vi "4145 Send Message.vi"(4 "source IN":string, 5 "status IN":bool[](array[boolean]), 7 "timeout ms":u32=25000, 8 "error in":T2, 9 "write mode (set END:0)":i32(ring) items=["send EOI with last character of string", "append CR to string and send EOI with CR", "append LF to string and send EOI with LF", "append CR LF to string and send EOI with LF", "append CR to string but do not send EOI", "append LF to string but do not send EOI", "append CR LF to string but do not send EOI", "do not send EOI"], 10 "write buffer IN":string, 11 "4145_GPIB_COM_IN":T1={"Address_string"="17", "timeout ms"=25000, "Terminator"=",", "LoggerQueue"=refnum}) -> (0 "error out":T2, 1 "status OUT":bool[](array[boolean]), 2 "byte count OUT":i32, 3 "4145_GPIB_COM_OUT":T1={"Address_string"="17", "timeout ms"=25000, "Terminator"=",", "LoggerQueue"=refnum})   [LabVIEW 2014]
doc: "Sends a string to a message based VXI instrument. In order to communicate with an instrument, you must first open the instrument by running the Open VXI Instrument or running the initialize VI (initialize VIs call the Open VXI Instrument in their block diagram). Use the instrument ID generated by the Open VXI Instrument to address the specific instrument, then set the write mode and enter the string to send. If a write error occurs, error code 1230 is returned. If you fail to open the instrument, error code 1232 is returned."
uses:
  typedef/4145_GPIB_Com.ctl
  typedef/4145_que_msg.ctl
  typedef/4145 command enum.ctl
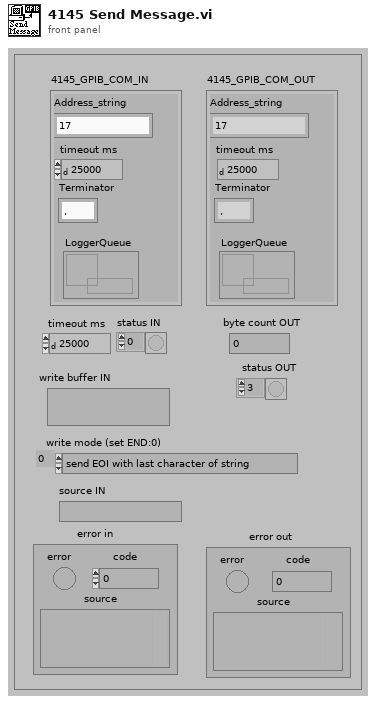
[diagram p1: front panel]
types:
  T1 = typedef "4145_GPIB_Com.ctl" = cluster{"Address_string":string, "timeout ms":u32, "Terminator":string, "LoggerQueue":refnum<queue>}
  T2 = cluster{"error":bool, "code":i32, "source":string}
  T3 = typedef "4145 command enum.ctl" = enum16{"DEFAULT", "INFORMATION", "ERROR", "STATUS", "CAUTION", "WARNING", "OFFLINE", "STOP"}
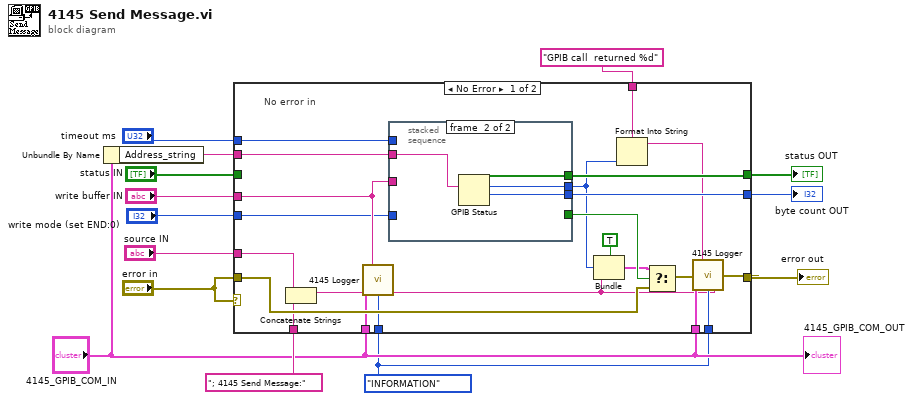
[diagram p0: block diagram]
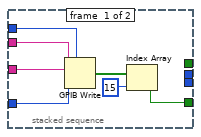
[diagram p2: hidden frame]
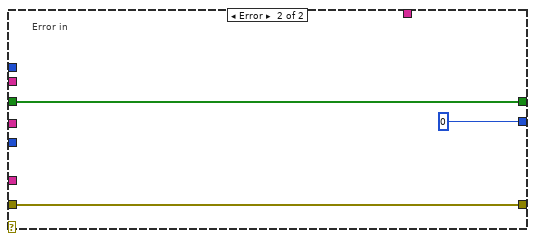
[diagram p3: hidden frame]
diagram:
  w2 = 4145_command_enum."INFORMATION" ("msg_type")
  n1 = Unbundle By Name("4145_GPIB_COM_IN") -> ("Address_string"=w10:string)
  n2 = case shown="No Error" "error in" {
    tunnel: "status IN" -> [_ w48]
    tunnel: [w33 w48] -> w13
    tunnel: [w16 w49] -> w11
    tunnel: "error in" -> [w32 w49]
    tunnel: [w34 0] -> w14
    tunnel: "4145_GPIB_COM_IN" -> [w31 _]
    tunnel: w10 -> [w30 _]
    tunnel: "write buffer IN" -> [w29 _]
    tunnel: w2 -> [w28 _]
    tunnel: "; 4145 Send Message:" -> [w27 _]
    tunnel: "timeout ms" -> [w26 _]
    tunnel: "write mode (set END:0)" -> [w25 _]
    tunnel: "source IN" -> [w24 _]
    tunnel: "4145_GPIB_COM_IN" -> [w23 _]
    tunnel: w2 -> [w22 _]
    tunnel: "GPIB call  returned %d" -> [w20 _]
    frame No Error {
      # "No error in"
      n3 = Concatenate Strings(w24, w27) -> (w21:string)
      n4 = call "4145 Logger.vi"("4145_GPIB_COM_ctrl"=w31, "msg"=w29, "msg_type"=w28, "origin vi"=w21) -> ()  [unwired: 11 in, 1 out]
      n5 = stacked-sequence {
        tunnel: [_ w46] -> w33
        tunnel: [_ w47] -> w34
        tunnel: [w40 _] -> w35
        tunnel: w25 -> [w37 _]
        tunnel: w29 -> [w41 _]
        tunnel: [_ w45] -> w19
        tunnel: w30 -> [w39 w44]
        tunnel: w26 -> [w38 _]
        frame #0 {
          n6 = GPIB Write(0:w39, 1:w41, 2:w37, 4:w38) -> (5:w42:bool[])  [unwired: 1 in, 1 out]
          n7 = Index Array(array=w42, index=15) -> (element=w40:bool)
        }
        frame #1 {
          n8 = GPIB Status(0:w44) -> (2:w46:bool[], 3:w45:i16, 4:w47:i32)  [unwired: 1 in, 1 out]
        }
      }
      n9 = Bundle(TRUE, "GPIB error"=w19, w21) -> (w15:cluster{bool, "GPIB error":i16, string})  [unwired: 1 in]
      n10 = Format Into String(format string=w20, w19) -> (resulting string=w18:string)  [unwired: 2 in, 1 out]
      n11 = Select(t=w15, s=w35, f=w32) -> (s? t:f=w17:T2)
      n12 = call "4145 Logger.vi"("4145_GPIB_COM_ctrl"=w23, "msg"=w18, "msg_type"=w22, "origin vi"=w21, "error in (no error)"=w17) -> ("error out"=w16:errorcluster)  [unwired: 10 in]
    }
    frame Error {
      # "Error in"
    }
  }
  "status OUT" <- w13
  "byte count OUT" <- w14
  "error out" <- w11
  "4145_GPIB_COM_OUT" <- "4145_GPIB_COM_IN"
